vi "sortSTDataByChannel.vi"(8 "error in (no error)":errorcluster, 9 "data":T2, 10 "channels":refnum<class "Channel.lvclass">[](array[class]), 11 "ScriptEventList in":refnum<class "ScriptEventList.lvclass">) -> (0 "error out":errorcluster, 2 "channelData":T1(array[cluster]), 3 "ScriptEventList out":refnum<class "ScriptEventList.lvclass">)   [LabVIEW 2011, in "Tools.lvlib" / "Scripting.lvlib" / "ScriptEventList.lvclass"]
uses:
  ScriptEventList.lvclass
  DatabaseHelpers/Database Objects/Channel/Channel.lvclass
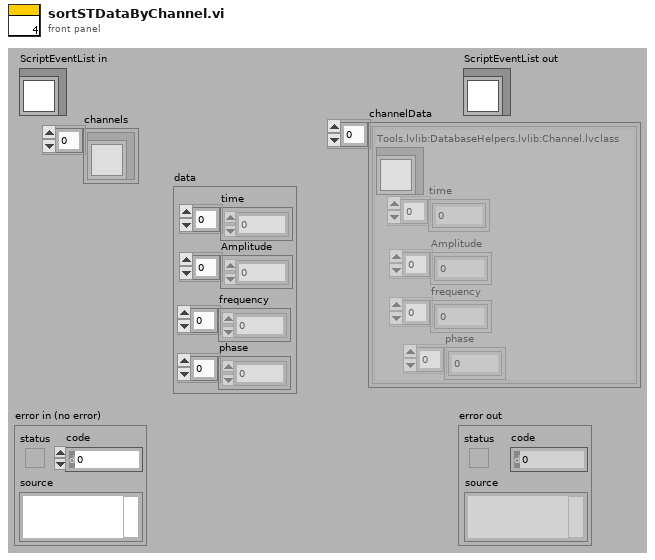
[diagram p1: front panel]
types:
  T1 = cluster{"Tools.lvlib:DatabaseHelpers.lvlib:Channel.lvclass":refnum<class "Channel.lvclass">, "time":dbl[], "Amplitude":dbl[], "frequency":dbl[], "phase":dbl[]}[]
  T2 = cluster{"time":dbl[], "Amplitude":dbl[], "frequency":dbl[], "phase":dbl[]}
  T3 = cluster{"Tools.lvlib:DatabaseHelpers.lvlib:Channel.lvclass":refnum<class "Channel.lvclass">, dbl[], dbl[], dbl[], dbl[]}
  T4 = cluster{"Channel.lvclass":refnum<class "Channel.lvclass">, "time":dbl[], "Amplitude":dbl[], "frequency":dbl[], "phase":dbl[]}[]
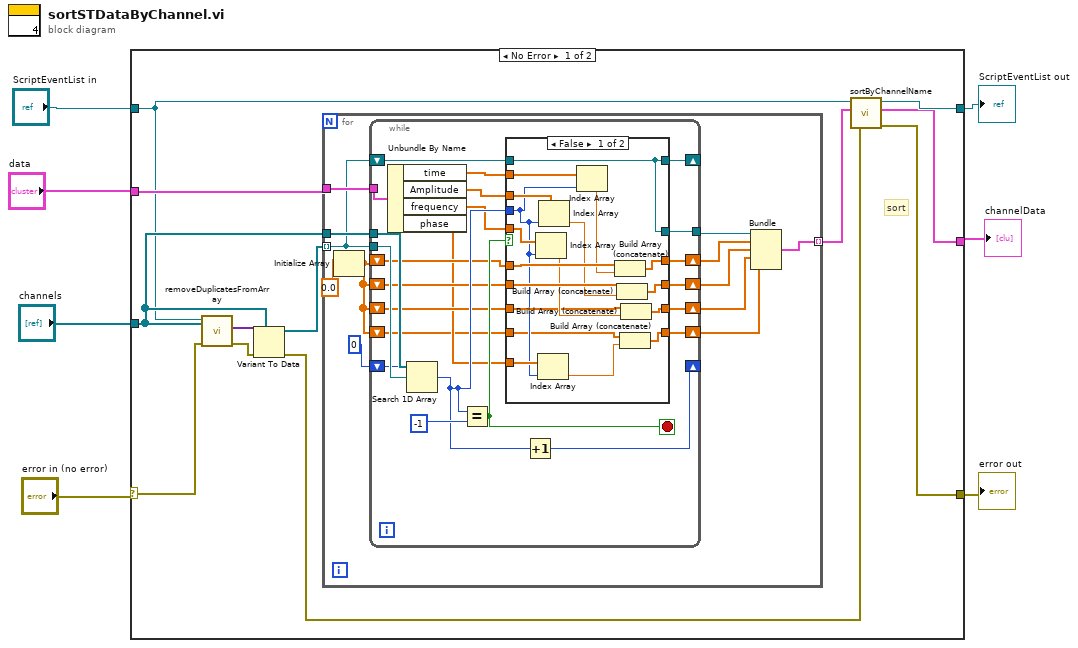
[diagram p0: block diagram]
diagram:
  n1 = case shown="No Error" "error in (no error)" {
    selector: "error in (no error)" -> [w16 w79]
    tunnel: [w10 w79] -> w5
    tunnel: [w12 w78] -> w6
    tunnel: "ScriptEventList in" -> [w13 w78]
    tunnel: "data" -> [w14 _]
    tunnel: "channels" -> [w17 _]
    tunnel: [w8 _] -> w1
    frame No Error {
      # "sort"
      n2 = call "removeDuplicatesFromArray.vi"("error in (no error)"=w16, "Array"=w17, "ScriptEventList in"=w13) -> ("error out"=w15:errorcluster, "Array out"=w19:variant[])  [unwired: 6 in, 1 out]
      n3 = Variant To Data(error in=w15, type=w17, Variant=w19) -> (data=w18:refnum<class "Channel.lvclass">[], error out=w11:errorcluster)
      n4 = for {
        tunnel: w14 -> [w29]
        tunnel: w17 -> [w31]
        tunnel: w18 -> [w27] mode=indexing
        tunnel: [w23] -> w9 mode=indexing
        n5 = Initialize Array(0.0) -> (w21:dbl[])  [unwired: 1 in]
        n6 = while {
          tunnel: w31 -> [w54]
          tunnel: w29 -> [w40]
          tunnel: w27 -> [w53]
          shift-right: [w49] -> _
          shift-left: 0 -> [w50]
          shift-right: [w47] -> w25
          shift-left: w21 -> [w46]
          shift-right: [w45] -> w24
          shift-left: w21 -> [w44]
          tunnel: [w43] -> w26
          shift-right: [w42] -> _
          shift-left: w27 -> [w41]
          shift-right: [w36] -> w22
          shift-left: w21 -> [w35]
          shift-right: [w32] -> w20
          shift-left: w21 -> [w33]
          stop <- w51 stop-if-true
          n7 = Unbundle By Name(w40) -> ("time"=w39:dbl[], "Amplitude"=w38:dbl[], "frequency"=w37:dbl[], "phase"=w34:dbl[])
          n8 = Search 1D Array(1D array=w54, element=w53, start index (0)=w50) -> (index of element=w48:i32)
          n9 = Equal?(x=w48, y=-1) -> (x = y?=w51:bool)
          n10 = case shown="False" w51 {
            tunnel: w48 -> [w59 _]
            tunnel: [w72 w77] -> w47
            tunnel: w46 -> [w71 w77]
            tunnel: [w70 w76] -> w45
            tunnel: w44 -> [w69 w76]
            tunnel: [w55 w75] -> w43
            tunnel: [w55 w75] -> w42
            tunnel: w41 -> [w55 w75]
            tunnel: w39 -> [w68 _]
            tunnel: w38 -> [w67 _]
            tunnel: w37 -> [w64 _]
            tunnel: [w62 w74] -> w36
            tunnel: w35 -> [w61 w74]
            tunnel: w34 -> [w60 _]
            tunnel: w33 -> [w58 w73]
            tunnel: [w56 w73] -> w32
            frame False {
              n11 = Index Array(array=w64, index=w59) -> (element=w63:dbl)
              n12 = Index Array(array=w60, index=w59) -> (element=w57:dbl)
              n13 = Index Array(array=w67, index=w59) -> (element=w65:dbl)
              n14 = Index Array(array=w68, index=w59) -> (element=w66:dbl)
              n15 = Build Array (concatenate)(w71, w66) -> (w72:dbl[])
              n16 = Build Array (concatenate)(w69, w65) -> (w70:dbl[])
              n17 = Build Array (concatenate)(w58, w57) -> (w56:dbl[])
              n18 = Build Array (concatenate)(w61, w63) -> (w62:dbl[])
            }
            frame True {
            }
          }
          n19 = Increment(x=w48) -> (x+1=w49:i32)
        }
        n20 = Bundle("Tools.lvlib:DatabaseHelpers.lvlib:Channel.lvclass"=w26, w25, w24, w22, w20) -> (w23:T3)  [unwired: 1 in]
      }
      n21 = call "sortByChannelName.vi"("error in (no error)"=w11, "channelData in"=w9, "ScriptEventList in"=w13) -> ("error out"=w10:errorcluster, "channelData"=w8:T4, "ScriptEventList out"=w12:refnum<class "ScriptEventList.lvclass">)  [unwired: 6 in]
    }
    frame Error {
    }
  }
  "error out" <- w5
  "ScriptEventList out" <- w6
  "channelData" <- w1
